vi "xijk_image_spectrum_analyzer.vi"(8 "error in (no error)":errorcluster, 11 "Start Path":path=path "H:/Programming/+ Labview/08 spectrum analyzer/example images/7666d8daad.jpg") -> (0 "error out":errorcluster, 2 "array out":dbl[][](array[numeric]), 3 "path out":path)   [LabVIEW 2009]
panel:
  out "yrange":dbl
  out "xrange":dbl
  out "ymax 2":i32
  out "ymin 2":i32
  out "xmax 2":i32
  out "xmin 2":i32
  in  "ymax":i32=1
  in  "ymin":i32
  in  "xmax":i32=1
  in  "xmin":i32
  in  "stop 2":bool
  in  "Zoom":sgl=1.0
  out "Image 3":T1(plugin-control)
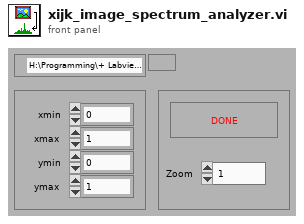
[diagram p1: front panel]
types:
  T1 = typedef "IMAQ Image.ctl" = refnum<image>
  T2 = typedef "ROI Descriptor" = cluster{"Global Rectangle":i32[], "Contours":cluster{"ID":enum32{"External", "Internal"}, "Type":u32, "Coordinates":i32[]}[]}
  T3 = cluster{"ID":enum32{"External", "Internal"}, "Type":u32, "Coordinates":i32[]}[]
  T4 = cluster{"ID":enum32{"External", "Internal"}, "Type":u32, "Coordinates":i32[]}
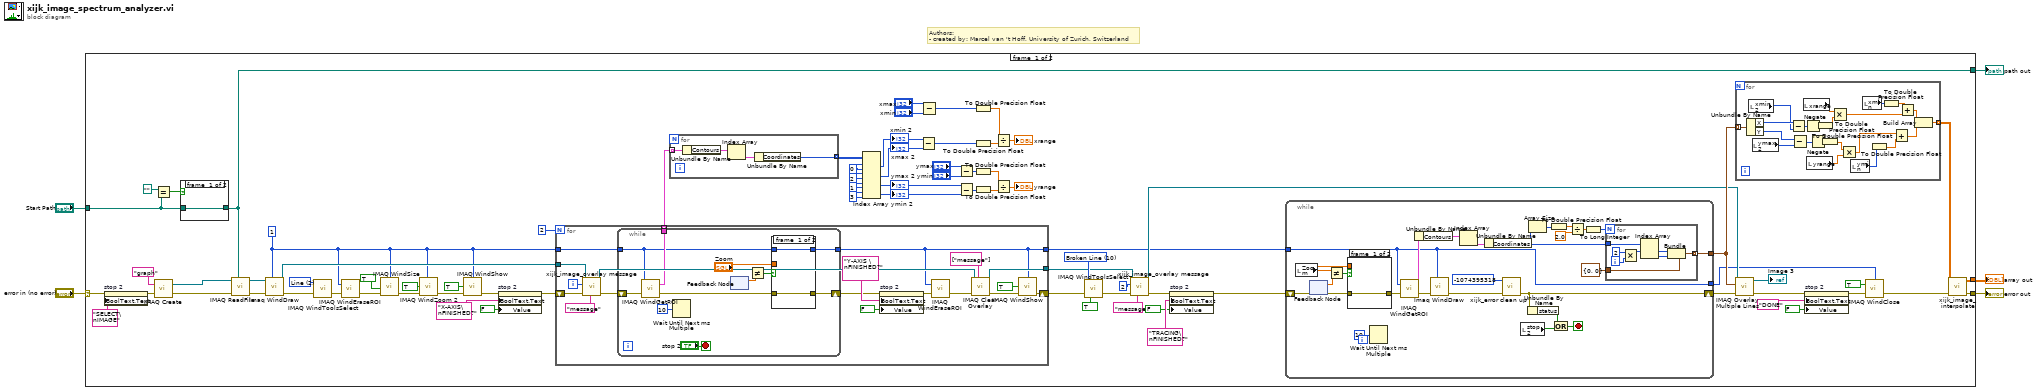
[diagram p0: block diagram]
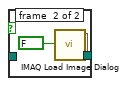
[diagram p2: hidden frame]
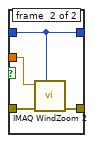
[diagram p3: hidden frame]
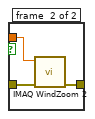
[diagram p4: hidden frame]
diagram:
  # "Authors: \n- created by: Marcel van 't Hoff, University of Zurich, Switzerland"
  n1 = case shown="No Error" "error in (no error)" {
    selector: "error in (no error)" -> [w14 w187]
    tunnel: [w52 w187] -> w5
    tunnel: [w51 _] -> w4
    tunnel: "Start Path" -> [w27 w186]
    tunnel: [w13 w186] -> w1
    frame #0 {
      w6 = 1 ("Window Number")
      w70 = 1 ("index (row)")
      w71 = 0 ("index (row)")
      w76 = u32 2 items=["No Selection", "Point", "Line", "Rectangle", "Oval", "Polygon", "Freehand Region", "Annulus", "Zoom", "Pan", "Broken Line", "Freehand Line", "Rotated Rectangle"] ("Tool (Point)")
      w81 = u32 10 items=["No Selection", "Point", "Line", "Rectangle", "Oval", "Polygon", "Freehand Region", "Annulus", "Zoom", "Pan", "Broken Line", "Freehand Line", "Rotated Rectangle"] ("Tool (Point)")
      n2 = property on="stop 2" class="Bool (strict)"(error in=w14, "BoolText.Text"="SELECT\nIMAGE" ("Boolean Text.Text")) -> (error out=w21:errorcluster)  [unwired: 1 in, 1 out]
      n3 = call "IMAQ Create"("Image Name"="graph", "error in (no error)"=w21) -> ("New Image"=w82:T1, "error out"=w48:errorcluster)  [unwired: 3 in]
      n4 = Equal?(x=path "", y=w27) -> (x = y?=w28:bool)
      n5 = case shown="False" w28 {
        tunnel: w27 -> [w84 _]
        tunnel: [w84 w85] -> w13
        frame #0 {
        }
        frame #1 {
          n6 = call "IMAQ Load Image Dialog"("Multiple Files? (No)"=FALSE) -> ("Path"=w85:path)  [unwired: 8 in, 2 out]
        }
      }
      n7 = call "IMAQ ReadFile"("File Path"=w13, "error in (no error)"=w48, "Image"=w82) -> ("error out"=w47:errorcluster, "Image Out"=w46:T1)  [unwired: 4 in, 3 out]
      n8 = call "Imaq WindDraw"("Window Number (0...15)"=w6, "error in (no error)"=w47, "Image"=w46) -> ("error out"=w77:errorcluster, "Image Out (duplicate)"=w20:T1)  [unwired: 7 in]
      n9 = call "IMAQ WindToolsSelect"("Tool (Point)"=w76, "error in (no error)"=w77) -> ("error out"=w50:errorcluster)  [unwired: 3 in, 1 out]
      n10 = call "IMAQ WindEraseROI"("Window Number"=w6, "error in (no error)"=w50) -> ("error out"=w49:errorcluster)  [unwired: 4 in]
      n11 = call "IMAQ WindSize"("error in (no error)"=w49, "Scrollbars? (N)"=TRUE, "Window Number"=w6) -> ("error out"=w31:errorcluster)  [unwired: 3 in, 2 out]
      n12 = call "IMAQ WindZoom 2"("Window Number (0...15)"=w6, "error in (no error)"=w31, "Zoom to Fit? (False)"=TRUE) -> ("error out"=w12:errorcluster)  [unwired: 5 in, 3 out]
      n13 = call "IMAQ WindShow"("error in (no error)"=w12, "Bring To Front? (N)"=TRUE, "Window Number (0...15)"=w6) -> ("error out"=w37:errorcluster)  [unwired: 3 in, 2 out]
      n14 = property on="stop 2" class="Bool (strict)"(error in=w37, "BoolText.Text"="X-AXIS\nFINISHED?" ("Boolean Text.Text"), "Value"=FALSE ("stop 2")) -> (error out=w36:errorcluster)  [unwired: 1 in, 1 out]
      n15 = for {
        N: 2 -> [_]
        tunnel: [w131] -> w74 mode=indexing
        tunnel: w20 -> [w129]
        tunnel: [w128] -> w42
        shift-right: [w124] -> w11
        shift-left: w36 -> [w117]
        tunnel: w6 -> [w114]
        tunnel: [w113] -> w9
        i -> [w130]
        n16 = call "xijk_image_overlay message.vi"("Group"="message", "error in"=w117, "message number"=w130, "Image In"=w129) -> ("error out"=w116:errorcluster, "Image Out (duplicate)"=w122:T1)  [unwired: 6 in]
        n17 = while {
          tunnel: [w139] -> w131
          shift-right: [w135] -> w119
          shift-left: w116 -> [w142]
          tunnel: w114 -> [w133]
          tunnel: [w132] -> w113
          stop <- "stop 2" stop-if-true
          n18 = call "IMAQ WindGetROI"("Window Number (0...15)"=w133, "error in (no error)"=w142) -> ("ROI Descriptor"=w139:T2, "error out"=w136:errorcluster)  [unwired: 3 in]
          n19 = Wait Until Next ms Multiple(millisecond multiple=u32 10) -> ()  [unwired: 1 out]
          n20 = feedback #1() -> (w138:sgl)  [unwired: 1 in]
          n21 = Not Equal?(x="Zoom", y=w138) -> (x != y?=w137:bool)
          n22 = case shown="False" w137 {
            tunnel: w136 -> [w144 w148]
            tunnel: [w144 w147] -> w135
            tunnel: "Zoom" -> [_ w146]
            tunnel: w133 -> [w143 w145]
            tunnel: [w143 w145] -> w132
            frame #0 {
            }
            frame #1 {
              n23 = call "IMAQ WindZoom 2"("Window Number (0...15)"=w145, "error in (no error)"=w148, "Zoom Factor"=w146) -> ("error out"=w147:errorcluster)  [unwired: 5 in, 3 out]
            }
          }
        }
        n24 = property on="stop 2" class="Bool (strict)"(error in=w119, "BoolText.Text"="Y-AXIS \nFINISHED?" ("Boolean Text.Text"), "Value"=FALSE ("stop 2")) -> (error out=w120:errorcluster)  [unwired: 1 in, 1 out]
        n25 = call "IMAQ WindEraseROI"("Window Number"=w113, "error in (no error)"=w120) -> ("error out"=w126:errorcluster)  [unwired: 4 in]
        n26 = call "IMAQ Clear Overlay"("Groups"=string[] ["message"], "error in (no error)"=w126, "Image"=w122) -> ("error out"=w125:errorcluster, "Image Out"=w128:T1)  [unwired: 7 in]
        n27 = call "IMAQ WindShow"("error in (no error)"=w125, "Bring To Front? (N)"=TRUE, "Window Number (0...15)"=w113) -> ("error out"=w124:errorcluster)  [unwired: 3 in, 2 out]
      }
      n28 = for {
        tunnel: w74 -> [w110] mode=indexing
        tunnel: [w109] -> w73 mode=indexing
        n29 = Unbundle By Name(w110) -> ("Contours"=w111:T3)
        n30 = Index Array(array=w111) -> (element=w112:T4)  [unwired: 1 in]
        n31 = Unbundle By Name(w112) -> ("Coordinates"=w109:i32[])
      }
      n32 = Index Array(array=w73, index (row) #1=w71, index (col) #1=w71, index (row) #2=w71, index (col) #2=2 ("disabled index (col)"), index (row) #3=w70, index (col) #3=w70, index (row) #4=w70, index (col) #4=3 ("disabled index (col)")) -> (element #1=w55:i32, element #2=w54:i32, element #3=w63:i32, element #4=w62:i32)
      "xmin 2" <- w55
      "xmax 2" <- w54
      "ymin 2" <- w62
      "ymax 2" <- w63
      n33 = Subtract(x=w55, y=w54) -> (x-y=w60:i32)
      n34 = Subtract(x="xmax", y="xmin") -> (x-y=w61:i32)
      n35 = Subtract(x="ymax", y="ymin") -> (x-y=w59:i32)
      n36 = Subtract(x=w63, y=w62) -> (x-y=w58:i32)
      n37 = To Double Precision Float(number=w61) -> (double precision float=w17:dbl)
      n38 = To Double Precision Float(number=w60) -> (double precision float=w18:dbl)
      n39 = To Double Precision Float(number=w59) -> (double precision float=w16:dbl)
      n40 = To Double Precision Float(number=w58) -> (double precision float=w15:dbl)
      n41 = Divide(x=w17, y=w18) -> (x/y=→"xrange":dbl)
      n42 = Divide(x=w16, y=w15) -> (x/y=→"yrange":dbl)
      n43 = call "IMAQ WindToolsSelect"("Tool (Point)"=w81, "Get/Set Status? (Set)"=TRUE, "error in (no error)"=w11) -> ("error out"=w44:errorcluster)  [unwired: 2 in, 1 out]
      n44 = call "xijk_image_overlay message.vi"("Group"="message", "error in"=w44, "message number"=2, "Image In"=w42) -> ("error out"=w34:errorcluster, "Image Out (duplicate)"=w43:T1)  [unwired: 6 in]
      n45 = property on="stop 2" class="Bool (strict)"(error in=w34, "BoolText.Text"="TRACING\nFINISHED?" ("Boolean Text.Text"), "Value"=FALSE ("stop 2")) -> (error out=w10:errorcluster)  [unwired: 1 in, 1 out]
      n46 = while {
        tunnel: [w162] -> w68
        shift-right: [w160] -> w79
        shift-left: w10 -> [w150]
        tunnel: w9 -> [w149]
        tunnel: [w149] -> w7
        stop <- w158 stop-if-true
        n47 = local read "Zoom"() -> (w154:sgl)
        n48 = feedback #2() -> (w156:sgl)  [unwired: 1 in]
        n49 = Not Equal?(x=w154, y=w156) -> (x != y?=w155:bool)
        n50 = case shown="True" w155 {
          tunnel: w150 -> [w174 w177]
          tunnel: [w174 w176] -> w157
          tunnel: w154 -> [_ w175]
          frame #0 {
          }
          frame #1 {
            n51 = call "IMAQ WindZoom 2"("error in (no error)"=w177, "Zoom Factor"=w175) -> ("error out"=w176:errorcluster)  [unwired: 6 in, 3 out]
          }
        }
        n52 = Wait Until Next ms Multiple(millisecond multiple=u32 10) -> ()  [unwired: 1 out]
        n53 = call "IMAQ WindGetROI"("Window Number (0...15)"=w149, "error in (no error)"=w157) -> ("ROI Descriptor"=w163:T2, "error out"=w153:errorcluster)  [unwired: 3 in]
        n54 = Unbundle By Name(w163) -> ("Contours"=w170:T3)
        n55 = call "Imaq WindDraw"("Window Number (0...15)"=w149, "error in (no error)"=w153) -> ("error out"=w161:errorcluster)  [unwired: 8 in, 1 out]
        n56 = Index Array(array=w170) -> (element=w169:T4)  [unwired: 1 in]
        n57 = Unbundle By Name(w169) -> ("Coordinates"=w168:i32[])
        n58 = call "xijk_error clean up.vi"("error in"=w161, "code in"=-1074395318) -> ("error out"=w160:errorcluster)  [unwired: 9 in]
        n59 = local read "stop 2"() -> (w152:bool)
        n60 = Unbundle By Name(w160) -> ("status"=w159:bool)
        n61 = Array Size(array=w168) -> (size(s)=w165:i32)
        n62 = To Double Precision Float(number=w165) -> (double precision float=w151:dbl)
        n63 = Or(x=w159, y=w152) -> (x .or. y?=w158:bool)
        n64 = Divide(x=w151, y=2.0 ("size(s)")) -> (x/y=w166:dbl)
        n65 = To Long Integer(number=w166) -> (32bit integer=w164:i32)
        n66 = for {
          N: w164 -> [_]
          tunnel: cluster{"X":i32, "Y":i32} {"X"=0, "Y"=0} ("Start Point") -> [w185]
          tunnel: [w184] -> w162 mode=indexing
          tunnel: w168 -> [w183]
          i -> [w181]
          n67 = Multiply(x=2, y=w181) -> (x*y=w179:i32)
          n68 = Index Array(array=w183, index #1=w179) -> (element #1=w182:i32, element #2=w178:i32)  [unwired: 1 in]
          n69 = Bundle(cluster=w185, "X"=w182, "Y"=w178) -> (w184:cluster{"X":i32, "Y":i32})
        }
      }
      n70 = for {
        tunnel: w68 -> [w105] mode=indexing
        tunnel: [w87] -> w53 mode=indexing
        n71 = Unbundle By Name(w105) -> ("X"=w108:i32, "Y"=w107:i32)
        n72 = local read "xmin 2"() -> (w99:i32)
        n73 = local read "ymax 2"() -> (w106:i32)
        n74 = Subtract(x=w108, y=w99) -> (x-y=w100:i32)
        n75 = Subtract(x=w107, y=w106) -> (x-y=w98:i32)
        n76 = local read "xrange"() -> (w104:dbl)
        n77 = Negate(x=w100) -> (-x=w96:i32)
        n78 = local read "yrange"() -> (w101:dbl)
        n79 = Negate(x=w98) -> (-x=w97:i32)
        n80 = To Double Precision Float(number=w96) -> (double precision float=w103:dbl)
        n81 = To Double Precision Float(number=w97) -> (double precision float=w102:dbl)
        n82 = Multiply(x=w104, y=w103) -> (x*y=w95:dbl)
        n83 = Multiply(x=w102, y=w101) -> (x*y=w90:dbl)
        n84 = local read "ymin"() -> (w91:i32)
        n85 = local read "xmin"() -> (w94:i32)
        n86 = To Double Precision Float(number=w91) -> (double precision float=w92:dbl)
        n87 = To Double Precision Float(number=w94) -> (double precision float=w93:dbl)
        n88 = Add(x=w90, y=w92) -> (x+y=w88:dbl)
        n89 = Add(x=w93, y=w95) -> (x+y=w89:dbl)
        n90 = Build Array(w89, w88) -> (w87:dbl[])
      }
      n91 = call "IMAQ Overlay Multiple Lines"("error in (no error)"=w79, "Line End Points"=w68, "Image"=w43) -> ("error out"=w24:errorcluster, "Image Out"=→"Image 3":T1)  [unwired: 7 in]
      n92 = property on="stop 2" class="Bool (strict)"(error in=w24, "BoolText.Text"="DONE" ("Boolean Text.Text"), "Value"=FALSE ("stop 2")) -> (error out=w23:errorcluster)  [unwired: 1 in, 1 out]
      n93 = call "IMAQ WindClose"("Window Number (0...15)"=w7, "Close All Windows (False)"=TRUE, "error in (no error)"=w23) -> ("error out"=w40:errorcluster)  [unwired: 3 in]
      n94 = call "xijk_image_interpolate.vi"("error in"=w40, "array in"=w53) -> ("error out"=w52:errorcluster, "array out"=w51:dbl[][])  [unwired: 8 in]
    }
    frame #1 {
    }
  }
  "error out" <- w5
  "array out" <- w4
  "path out" <- w1
